vi "Obtain Stream.vi"(8 "error in (no error)":errorcluster, 11 "Name":string) -> (0 "error out":errorcluster, 3 "stream out":refnum<queue>)   [LabVIEW 2015, in "Sprocket.lvlib"]
uses:
  lib/Sprocket.lvlib
  Action/Action.ctl
  Action/Action Name.ctl
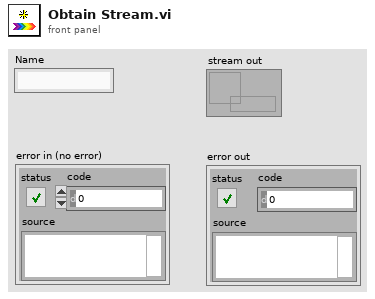
[diagram p1: front panel]
types:
  T1 = typedef "Sprocket.lvlib/Action.ctl" = cluster{"Name":T2, "Priority":i32, "Data":variant}
  T2 = typedef "Sprocket.lvlib/Action Name.ctl" = enum16{"No Action", "Drive Left", "Drive Right", "Drive Both", "Collector Spin"}
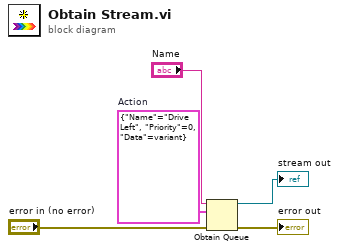
[diagram p0: block diagram]
diagram:
  w2 = T1 {"Name"=enum."Drive Left", "Priority"=0, "Data"=variant}  # Action
  n1 = Obtain Queue(name (unnamed)="Name", element data type=w2, error in (no error)="error in (no error)") -> (queue out=→"stream out":refnum<queue>, error out=→"error out":errorcluster)  [unwired: 2 in, 1 out]
